vi "RDADailyWIP.vi"() -> ()   [LabVIEW 2012]
uses:
  <vilib>/addons/database/Auxilliary.llb/DB Tools Cursor Type.ctl
  <vilib>/Utility/NIReport.llb/NI_report.lvclass
  <vilib>/addons/database/Connection.llb/DB Tools Open Connec (Path).vi
  <vilib>/addons/database/Connection.llb/Conn Execute.vi
  <vilib>/addons/database/Recordset.llb/Rec Fetch Recordset Data (R).vi
  <vilib>/addons/database/Recordset.llb/Rec Destroy - Connection.vi
  <vilib>/addons/database/Recordset.llb/Rec Fetch Integer Data (R).vi
  <vilib>/Utility/NIReport.llb/Append Text Table to Report (wrap).vi
  <vilib>/addons/database/_DB Variant To Data/Database Variant To Data.xnode
  <vilib>/addons/database/NI_Database_API.lvlib
  <vilib>/Utility/NIReport.llb/Excel/NI_Excel.lvclass
panel:
  out "error out":errorcluster
  in  "template (empty)":path=path "O:/Monitor/Report/SunplusWIP.xls"
  out "error out 2":errorcluster
  out "array":string[][](array[string])
  out "appended array":string[](array[string])
  out "recordset data":variant[][](array[variant])
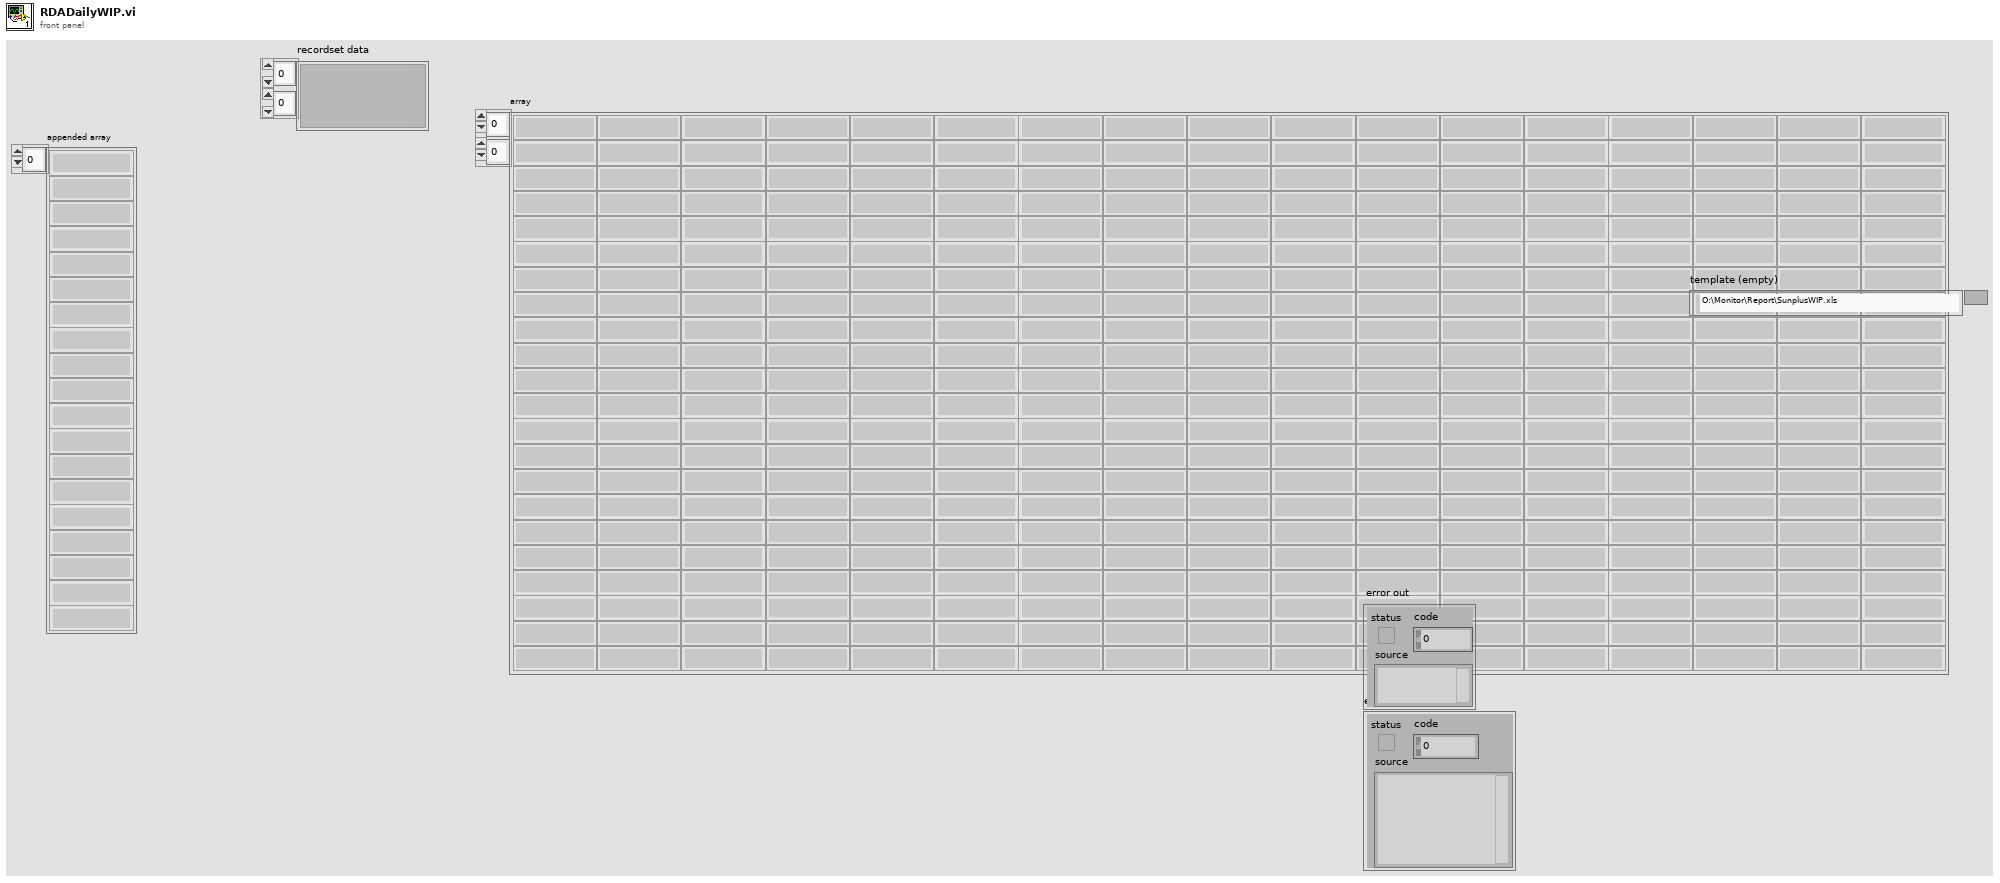
[diagram p1: front panel]
types:
  T1 = typedef "NI_Database_API.lvlib/DB Tools Cursor Type.ctl" = enum16{"forward-only", "keyset", "dynamic", "static"}
  T2 = typedef "NI_Database_API.lvlib/Conn ObjectReference.ctl" = refnum<k1>
  T3 = typedef "NI_Database_API.lvlib/Rec ObjectReference.ctl" = refnum<k1>
  T4 = enum16{"Standard Report", "HTML", "Word", "Excel"}
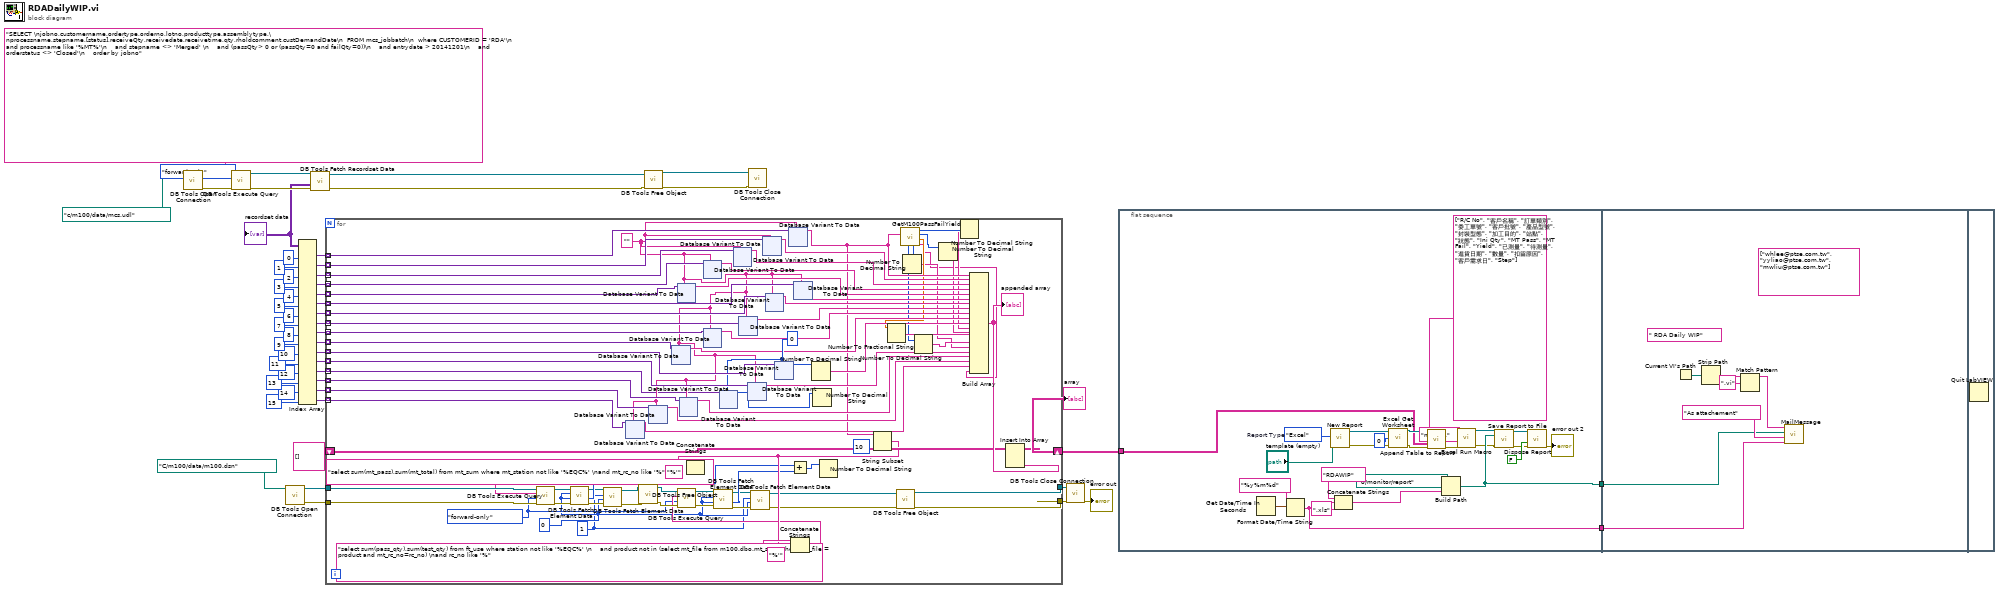
[diagram p0: block diagram]
diagram:
  n1 = call-poly <vilib>:"DB Tools Open Connection.vi"("connection information"=path "c:/m100/data/mcs.udl") -> ("error out"=w52:errorcluster, "connection reference"=w53:T2)  [unwired: 7 in]
  n2 = call-poly <vilib>:"DB Tools Execute Query.vi"("error in (no error)"=w52, "cursor type"=DB_Tools_Cursor_Type."forward-only", "SQL query"="SELECT \njobno,customername,ordertype,orderno,lotno,producttype,assemblytype,\nprocessname,stepname,[status],receiveQty,receivedate,receivetime,qty,rholdcomment,custDemandDate\n  FROM mcs_jobbatch\n  where CUSTOMERID = 'RDA'\n    and processname like '%MT%'\n    and stepname <> 'Merged' \n    and (passQty> 0 or (passQty=0 and failQty=0))\n    and entrydate > 20141201\n    and orderstatus <> 'Closed'\n    order by jobno", "connection reference"=w53) -> ("error out"=w50:errorcluster, "recordset reference"=w51:T3)  [unwired: 4 in]
  n3 = call-poly <vilib>:"DB Tools Open Connection.vi"("connection information"=path "C:/m100/data/m100.dsn") -> ("error out"=w6:errorcluster, "connection reference"=w7:T2)  [unwired: 7 in]
  n4 = call-poly <vilib>:"DB Tools Fetch Recordset Data.vi"("error in (no error)"=w50, "recordset reference"=w51) -> ("error out"=w48:errorcluster, "recordset data"=w42:variant[][], "recordset reference out"=w49:T3)  [unwired: 3 in]
  "recordset data" <- w42
  n5 = Index Array(array=w42, index (col) #1=0 ("disabled index (col)"), index (col) #2=1 ("index (col)"), index (col) #3=2 ("index (col)"), index (col) #4=3 ("index (col)"), index (col) #5=4 ("index (col)"), index (col) #6=5 ("index (col)"), index (col) #7=6 ("index (col)"), index (col) #8=7 ("index (col)"), index (col) #9=8 ("index (col)"), index (col) #10=9 ("index (col)"), index (col) #11=10 ("index (col)"), index (col) #12=11 ("index (col)"), index (col) #13=12 ("index (col)"), index (col) #14=13 ("index (col)"), index (col) #15=14 ("index (col)"), index (col) #16=15 ("index (col)")) -> (element #1=w25:variant[], element #2=w24:variant[], element #3=w23:variant[], element #4=w22:variant[], element #5=w21:variant[], element #6=w20:variant[], element #7=w19:variant[], element #8=w18:variant[], element #9=w17:variant[], element #10=w16:variant[], element #11=w15:variant[], element #12=w14:variant[], element #13=w13:variant[], element #14=w12:variant[], element #15=w11:variant[], element #16=w9:variant[])  [unwired: 16 in]
  n6 = for {
    tunnel: w25 -> [w135] mode=indexing
    tunnel: w24 -> [w134] mode=indexing
    tunnel: w23 -> [w133] mode=indexing
    tunnel: w22 -> [w132] mode=indexing
    tunnel: w21 -> [w131] mode=indexing
    tunnel: w20 -> [w130] mode=indexing
    tunnel: w19 -> [w129] mode=indexing
    tunnel: w18 -> [w128] mode=indexing
    tunnel: w17 -> [w127] mode=indexing
    tunnel: w16 -> [w126] mode=indexing
    tunnel: w15 -> [w125] mode=indexing
    tunnel: w14 -> [w124] mode=indexing
    tunnel: w13 -> [w81] mode=indexing
    tunnel: w12 -> [w123] mode=indexing
    tunnel: w11 -> [w122] mode=indexing
    shift-right: [w108] -> w3
    shift-left: string[][] [] ("array") -> [w107]
    tunnel: w9 -> [w106] mode=indexing
    tunnel: w7 -> [w104]
    tunnel: w6 -> [w103]
    tunnel: [w91] -> w5
    tunnel: [w90] -> w4
    w67 = 1
    w85 = DB_Tools_Cursor_Type."forward-only" ("cursor type")
    w68 = 0
    w121 = 0
    w105 = ""
    n7 = xnode "Database Variant To Data"("database variant"=w106, "type"=w105) -> ("data"=w80:string)  [unwired: 1 in, 1 out]
    n8 = xnode "Database Variant To Data"("database variant"=w122, "type"=w105) -> ("data"=w79:string)  [unwired: 1 in, 1 out]
    n9 = xnode "Database Variant To Data"("database variant"=w126, "type"=w105) -> ("data"=w112:string)  [unwired: 1 in, 1 out]
    n10 = xnode "Database Variant To Data"("database variant"=w131, "type"=w105) -> ("data"=w117:string)  [unwired: 1 in, 1 out]
    n11 = xnode "Database Variant To Data"("database variant"=w123, "type"=w105) -> ("data"=w78:string)  [unwired: 1 in, 1 out]
    n12 = xnode "Database Variant To Data"("database variant"=w132, "type"=w105) -> ("data"=w118:string)  [unwired: 1 in, 1 out]
    n13 = xnode "Database Variant To Data"("database variant"=w127, "type"=w105) -> ("data"=w113:string)  [unwired: 1 in, 1 out]
    n14 = xnode "Database Variant To Data"("database variant"=w81, "type"=w121) -> ("data"=w110:i32)  [unwired: 1 in, 1 out]
    n15 = xnode "Database Variant To Data"("database variant"=w133, "type"=w105) -> ("data"=w119:string)  [unwired: 1 in, 1 out]
    n16 = xnode "Database Variant To Data"("database variant"=w128, "type"=w105) -> ("data"=w114:string)  [unwired: 1 in, 1 out]
    n17 = xnode "Database Variant To Data"("database variant"=w124, "type"=w105) -> ("data"=w77:string)  [unwired: 1 in, 1 out]
    n18 = xnode "Database Variant To Data"("database variant"=w134, "type"=w105) -> ("data"=w120:string)  [unwired: 1 in, 1 out]
    n19 = xnode "Database Variant To Data"("database variant"=w129, "type"=w105) -> ("data"=w115:string)  [unwired: 1 in, 1 out]
    n20 = xnode "Database Variant To Data"("database variant"=w125, "type"=w121) -> ("data"=w111:i32)  [unwired: 1 in, 1 out]
    n21 = xnode "Database Variant To Data"("database variant"=w135, "type"=w105) -> ("data"=w66:string)  [unwired: 1 in, 1 out]
    n22 = xnode "Database Variant To Data"("database variant"=w130, "type"=w105) -> ("data"=w116:string)  [unwired: 1 in, 1 out]
    n23 = Number To Decimal String(number=w111) -> (decimal integer string=w97:string)  [unwired: 1 in]
    n24 = Number To Decimal String(number=w110) -> ()  [unwired: 1 in, 1 out]
    n25 = String Subset(string=w66, length (rest)=10 ("length (rest)")) -> (substring=w88:string)  [unwired: 1 in]
    n26 = Concatenate Strings("select sum(mt_pass),sum(mt_total) from mt_sum where mt_station not like '%EQC%' \nand mt_rc_no like '%" ("SQL query"), w88, "%'" ("string")) -> (w98:string)
    n27 = call-poly <vilib>:"DB Tools Execute Query.vi"("error in (no error)"=w103, "cursor type"=w85, "SQL query"=w98, "connection reference"=w104) -> ("error out"=w101:errorcluster, "recordset reference"=w102:T3)  [unwired: 4 in]
    n28 = call-poly <vilib>:"DB Tools Fetch Element Data.vi"("error in (no error)"=w101, "type"=w68, "column index"=w68, "recordset reference"=w102) -> ("error out"=w74:errorcluster, "data"=w83:i32, "recordset reference out"=w76:T3)  [unwired: 3 in]
    n29 = call-poly <vilib>:"DB Tools Fetch Element Data.vi"("error in (no error)"=w74, "type"=w68, "column index"=w67, "recordset reference"=w76) -> ("error out"=w73:errorcluster, "recordset reference out"=w75:T3)  [unwired: 3 in, 1 out]
    n30 = call-poly <vilib>:"DB Tools Free Object.vi"("error in (no error)"=w73, "recordset reference"=w75) -> ("error out"=w94:errorcluster, "connection reference"=w95:T2)  [unwired: 8 in]
    n31 = Concatenate Strings("select sum(pass_qty),sum(test_qty) from ft_use where station not like '%EQC%' \n    and product not in (select mt_file from m100.dbo.mt_sum where mt_file = product and mt_rc_no=rc_no) \nand rc_no like '%" ("SQL query"), w88, "%'" ("string")) -> (w86:string)
    n32 = call-poly <vilib>:"DB Tools Execute Query.vi"("error in (no error)"=w94, "cursor type"=w85, "SQL query"=w86, "connection reference"=w95) -> ("error out"=w92:errorcluster, "recordset reference"=w93:T3)  [unwired: 4 in]
    n33 = call-poly <vilib>:"DB Tools Fetch Element Data.vi"("error in (no error)"=w92, "type"=w68, "column index"=w68, "recordset reference"=w93) -> ("error out"=w70:errorcluster, "data"=w82:i32, "recordset reference out"=w72:T3)  [unwired: 3 in]
    n34 = call-poly <vilib>:"DB Tools Fetch Element Data.vi"("error in (no error)"=w70, "type"=w68, "column index"=w67, "recordset reference"=w72) -> ("error out"=w69:errorcluster, "recordset reference out"=w71:T3)  [unwired: 3 in, 1 out]
    n35 = Add(x=w83, y=w82) -> (x+y=w84:i32)
    n36 = Number To Decimal String(number=w84) -> ()  [unwired: 1 in, 1 out]
    n37 = call-poly <vilib>:"DB Tools Free Object.vi"("error in (no error)"=w69, "recordset reference"=w71) -> ("error out"=w90:errorcluster, "connection reference"=w91:T2)  [unwired: 8 in]
    n38 = call "GetM100PassFailYield.vi"("RCNO"=w66) -> ("Step"=w55:string, "Yield"=w61:dbl, "Fail"=w63:i32, "Pass"=w65:i32, "待測"=w59:i32, "已測"=w58:i32)  [unwired: 5 in]
    n39 = Number To Fractional String(number=w61) -> (F-format string=w60:string)  [unwired: 3 in]
    n40 = Number To Decimal String(number=w59) -> (decimal integer string=w56:string)  [unwired: 1 in]
    n41 = Number To Decimal String(number=w58) -> (decimal integer string=w57:string)  [unwired: 1 in]
    n42 = Number To Decimal String(number=w63) -> (decimal integer string=w62:string)  [unwired: 1 in]
    n43 = Number To Decimal String(number=w65) -> (decimal integer string=w64:string)  [unwired: 1 in]
    n44 = Build Array(w66, w120, w119, w118, w117, w116, w115, w114, w113, w112, w97, w64, w62, w60, w57, w56, w77, w78, w79, w80, w55) -> (w109:string[])
    "appended array" <- w109
    n45 = Insert Into Array(array=w107, new element=w109) -> (w108:string[][])  [unwired: 2 in]
  }
  "array" <- w3
  n46 = call-poly <vilib>:"DB Tools Free Object.vi"("error in (no error)"=w48, "recordset reference"=w49) -> ("error out"=w46:errorcluster, "connection reference"=w47:T2)  [unwired: 8 in]
  n47 = call <vilib>:"DB Tools Close Connection.vi"("error in (no error)"=w46, "connection reference"=w47) -> ()  [unwired: 5 in, 1 out]
  n48 = call <vilib>:"DB Tools Close Connection.vi"("error in (no error)"=w4, "connection reference"=w5) -> ("error out"=→"error out":errorcluster)  [unwired: 5 in]
  n49 = flat-sequence {
    tunnel: w3 -> [w656]
    tunnel: [w655] -> w54
    tunnel: [w648] -> w1
    tunnel: w54 -> [w675]
    tunnel: w1 -> [w674]
    frame #0 {
      w673 = T4."Excel"  # Report Type
      n50 = Get Date/Time In Seconds() -> (seconds since 1Jan1904=w660:timestamp)
      n51 = Format Date/Time String(time format string (%c)="%y%m%d", seconds (now)=w660) -> (date/time string=w648:string)  [unwired: 1 in]
      n52 = call <vilib>:"New Report.vi"("report type"=w673, "template (empty)"="template (empty)") -> ("report out"=w672:refnum<class "NI_report.lvclass">, "error out"=w671:errorcluster)  [unwired: 12 in]
      n53 = Concatenate Strings("RDAWIP" ("string"), w648, ".xls" ("string")) -> (w661:string)
      n54 = call <vilib>:"Excel Get Worksheet.vi"("report in"=w672, "worksheet index (0)"=0, "error in (no error)"=w671) -> ("report out"=w668:refnum<class "NI_report.lvclass">, "error out"=w667:errorcluster)  [unwired: 11 in]
      n55 = call-poly <vilib>:"Append Table to Report.vi"("report in"=w668, "column headers"=string[] ["R/C No", "客戶名稱", "訂單類別", "委工單號", "客戶批號", "產品型號", "封裝型態", "加工目的", "站點", "狀態", "Ini Qty", "MT Pass", "MT Fail", "Yield", "已測量", "待測量", "進貨日期", "數量", "扣留原因", "客戶需求日", "Step"], "text data"=w656, "error in (no error)"=w667) -> ("report out"=w651:refnum<class "NI_report.lvclass">, "error out"=w654:errorcluster)  [unwired: 8 in, 2 out]
      n56 = Build Path(base path=path "o:/monitor/report", name or relative path=w661) -> (appended path=w655:path)
      n57 = call <vilib>:"Excel Run Macro.vi"("report in"=w651, "macro name"="macro1", "error in (no error)"=w654) -> ("report out"=w653:refnum<class "NI_report.lvclass">, "error out"=w652:errorcluster)  [unwired: 10 in, 1 out]
      n58 = call-dynamic "Save Report to File.vi"("report in"=w653, "report file path"=w655, "error in (no error)"=w652) -> ("report out"=w665:refnum<class "NI_report.lvclass">, "error out"=w664:errorcluster)  [unwired: 11 in]
      n59 = call-dynamic "Dispose Report.vi"("report in"=w665, "save changes? (F)"=FALSE, "error in (no error)"=w664) -> ("error out"=→"error out 2":errorcluster)  [unwired: 12 in]
    }
    frame #1 {
      (unwired) string[] ["whlee@ptse.com.tw", "yyliao@ptse.com.tw", "mwliu@ptse.com.tw"] ("recipients")
      (unwired) " RDA Daily WIP" ("subject ([No Subject])")
      n60 = Current VI's Path() -> (path=w680:path)
      n61 = Strip Path(path=w680) -> (name=w679:string)  [unwired: 1 out]
      n62 = Match Pattern(string=w679, regular expression=".vi") -> (before substring=w677:string)  [unwired: 1 in, 3 out]
      n63 = call "MailMessage.vi"("AddSubject"=w674, "message"="As attachement", "file path"=w675, "program"=w677) -> ()  [unwired: 8 in]
    }
    frame #2 {
      n64 = Quit LabVIEW() -> ()  [unwired: 1 in]
    }
  }
